vi "GDSString_XML_GetTags.vi"(1 "XML LV data in":string, 3 "FilterTags(Only these tags, ignored if not wired)":string, 5 "error in (no error)":errorcluster) -> (15 "Tags":string[](array[string]), 16 "Values":string[](array[string]), 17 "Attributes":string[](array[string]), 19 "error out":errorcluster)   [LabVIEW 2020]
doc: "Reads an XML tag."
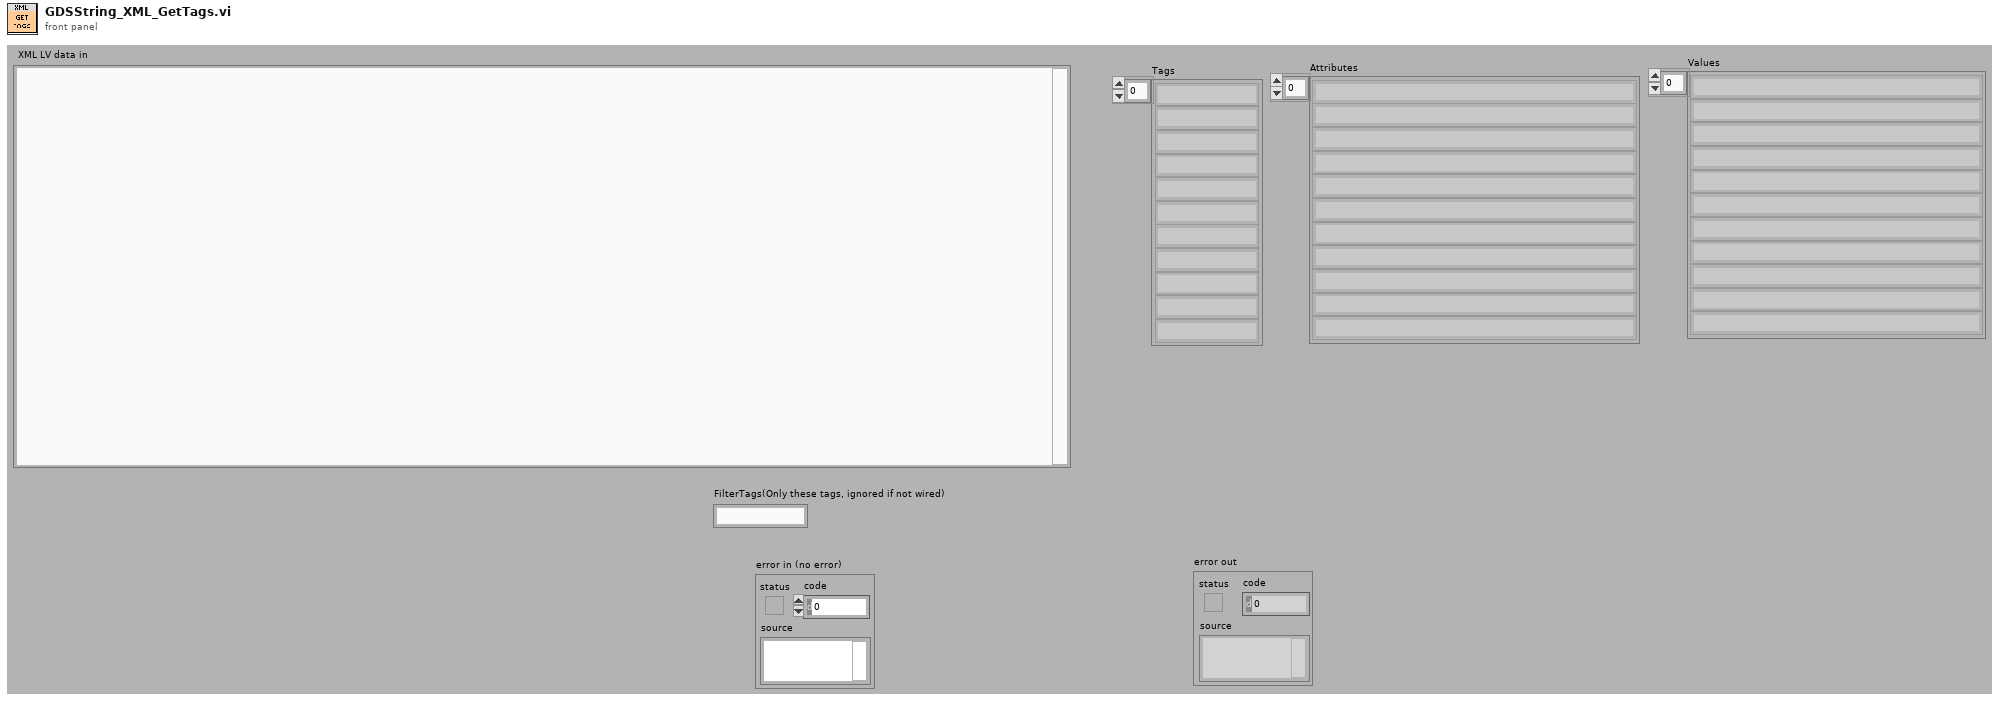
[diagram p1: front panel]
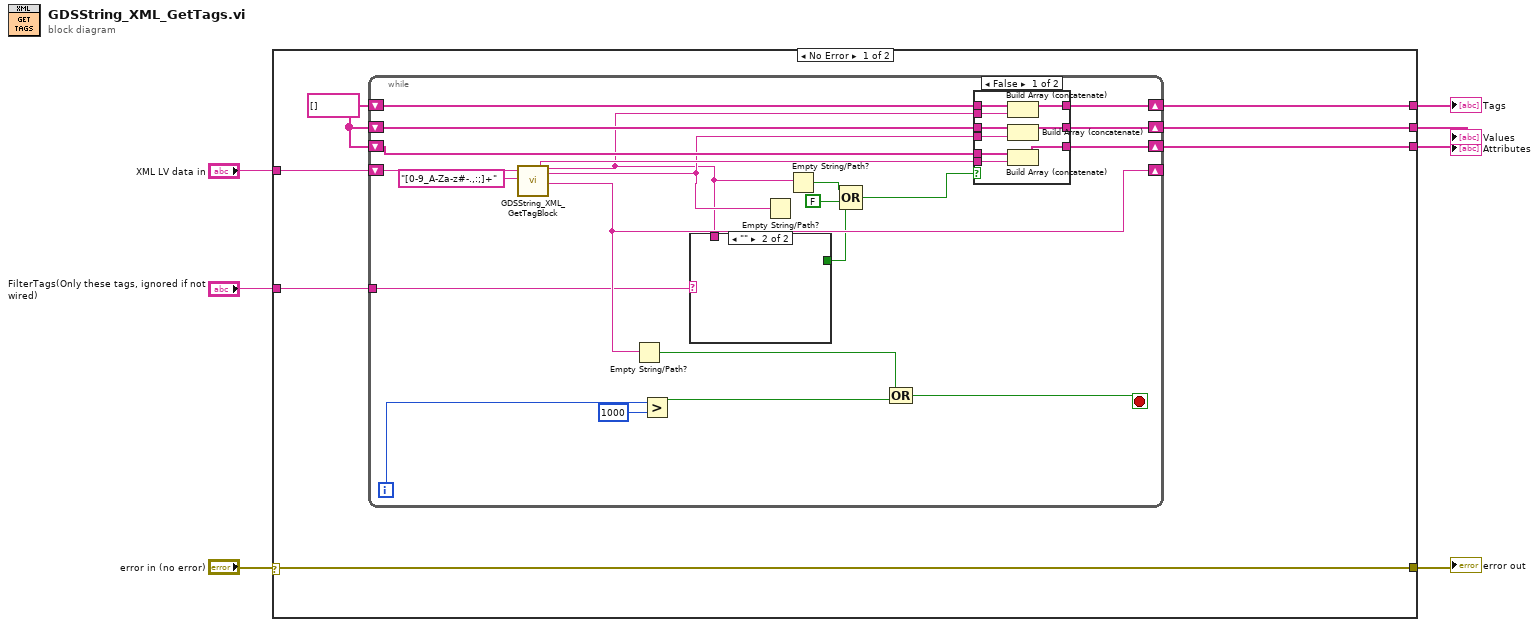
[diagram p0: block diagram]
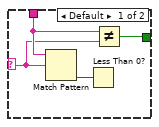
[diagram p2: hidden frame]
diagram:
  n1 = case shown="No Error" "error in (no error)" {
    selector: "error in (no error)" -> [w11 w53]
    tunnel: [w11 w53] -> w7
    tunnel: "XML LV data in" -> [w14 _]
    tunnel: [w13 _] -> w5
    tunnel: [w12 _] -> w4
    tunnel: [w9 _] -> w2
    tunnel: "FilterTags(Only these tags, ignored if not wired)" -> [w8 _]
    frame No Error {
      w10 = string[] []
      n2 = while {
        shift-right: [w29] -> _
        shift-left: w14 -> [w31]
        shift-right: [w35] -> w13
        shift-left: w10 -> [w36]
        shift-right: [w33] -> w12
        shift-left: w10 -> [w34]
        shift-right: [w23] -> w9
        shift-left: w10 -> [w24]
        tunnel: w8 -> [w17]
        i -> [w27]
        stop <- w32 stop-if-true
        n3 = call <resource>:"GDSString_XML_GetTagBlock.vi"("TextIn"=w31, "TagName"="[0-9_A-Za-z#-.,:;]+") -> ("AttributeString"=w22:string, "TagName"=w18:string, "TextWithinTag"=w21:string, "TextAfterTag"=w29:string)  [unwired: 11 in, 3 out]
        n4 = Empty String/Path?(string/path=w29) -> (empty?=w28:bool)
        n5 = Greater?(x=w27, y=1000) -> (0:w25:bool)
        n6 = case shown="\"\"" w17 {
          selector: w17 -> [w38 _]
          tunnel: w18 -> [w39 _]
          tunnel: [w37 _] -> w16
          frame Default {
            n7 = Match Pattern(string=w39, regular expression=w38) -> (offset past match=w40:i32)  [unwired: 4 out]
            n8 = Less Than 0?(x=w40) -> ()  [unwired: 1 out]
            n9 = Not Equal?(x=w39, y=w38) -> (x != y?=w37:bool)
          }
          frame "" {
          }
        }
        n10 = Empty String/Path?(string/path=w21) -> ()  [unwired: 1 out]
        n11 = Empty String/Path?(string/path=w18) -> (empty?=w20:bool)
        n12 = Compound Arithmetic op=OR(w20, FALSE ("value"), w16) -> (w19:bool)
        n13 = Compound Arithmetic op=OR(w28, w25) -> (w32:bool)
        n14 = case shown="False" w19 {
          tunnel: w36 -> [w49 w52]
          tunnel: w18 -> [w48 _]
          tunnel: [w47 w52] -> w35
          tunnel: w34 -> [w46 w51]
          tunnel: [w44 w51] -> w33
          tunnel: w21 -> [w45 _]
          tunnel: w24 -> [w43 w50]
          tunnel: [w42 w50] -> w23
          tunnel: w22 -> [w41 _]
          frame False {
            n15 = Build Array (concatenate)(w49, w48) -> (w47:string[])
            n16 = Build Array (concatenate)(w46, w45) -> (w44:string[])
            n17 = Build Array (concatenate)(w43, w41) -> (w42:string[])
          }
          frame True {
          }
        }
      }
    }
    frame Error {
    }
  }
  "error out" <- w7
  "Tags" <- w5
  "Values" <- w4
  "Attributes" <- w2
